vi "RT.vi"() -> ()   [LabVIEW 2020]
uses:
  <vilib>/FPGAPlugInAG/cRIO-9054/niLvFpga_Open_cRIO-9054.vi
  <vilib>/FPGAPlugInAG/cRIO-9054/niLvFpga_Reset_cRIO-9054.vi
  <vilib>/Utility/error.llb/Error Cluster From Error Code.vi
  <vilib>/rvi/errors/niLvFpgaAdjustHostInterfaceError.vi
  <vilib>/FPGAPlugInAG/cRIO-9054/niLvFpga_Run_cRIO-9054.vi
  <vilib>/FPGAPlugInAG/cRIO-9054/niLvFpga_Close_cRIO-9054.vi
  <vilib>/rvi/interface/nirviOpenFPGA/nirviOpenFPGA.xnode
  FPGA Bitfiles/fftwithlatch_FPGATarget_FPGA_RWnWaooWQ68.lvbitx
  FPGA.vi
  <vilib>/rvi/interface/nirviMethod/nirviMethod.xnode
  <vilib>/rvi/interface/nirviReadWriteControl/nirviReadWriteControl.xnode
  <vilib>/rvi/interface/nirviCloseFPGA/nirviCloseFPGA.xnode
  <vilib>/rvi/errors/niLvFpgaMergeErrorWithErrorCode.vi
  <vilib>/FPGAPlugInAG/cRIO-9054/niLvFpga_ReadFifo_cRIO-9054.vi
  NiFpgaLv.dll
  <vilib>/FPGAPlugInAG/cRIO-9054/niLvFpga_StartFifo_cRIO-9054.vi
panel:
  out "index":i32[](array[numeric])
  out "Index":i32[](graph)
  out "IMG":dbl[](graph)
  out "REAL":dbl[](graph)
  in  "FFT loop iterations":i32
  in  "auto stop":bool=TRUE
  out "FFT time (uSec)":u32
  out "data collection time (uSec)":u32
  in  "number of date points":i32=9000
  out "Timed Out?":bool
  in  "requested Loop rate (Hz)":u32=1000
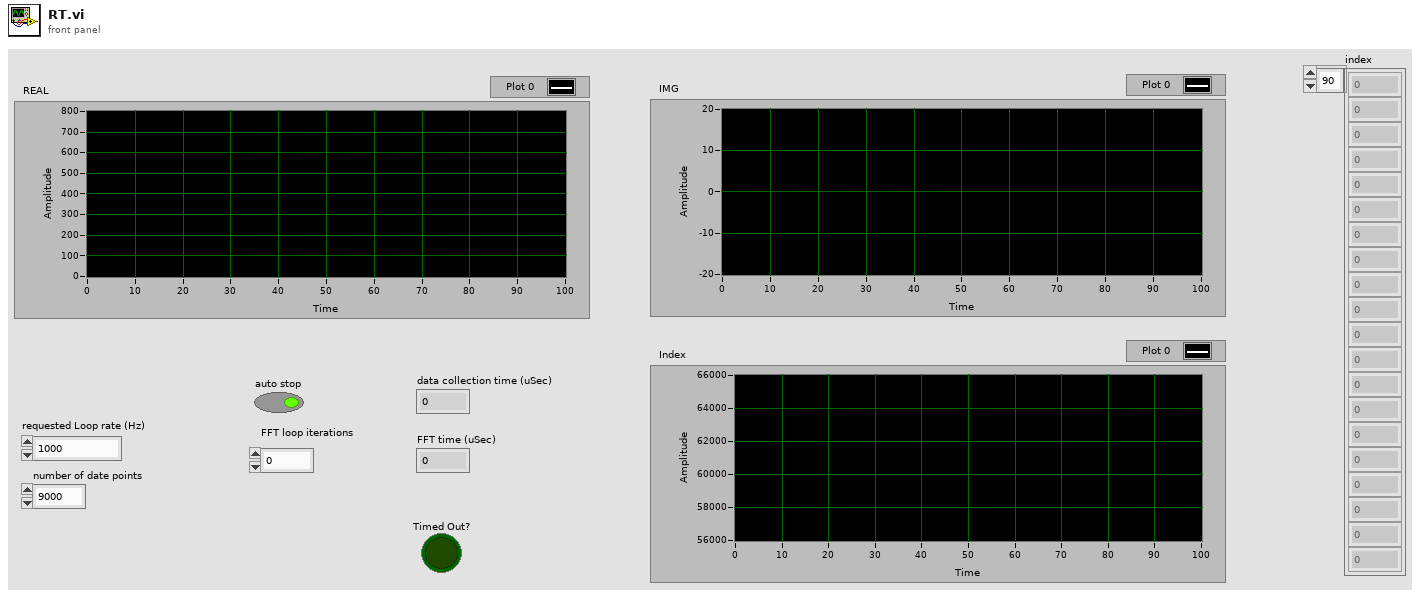
[diagram p1: front panel]
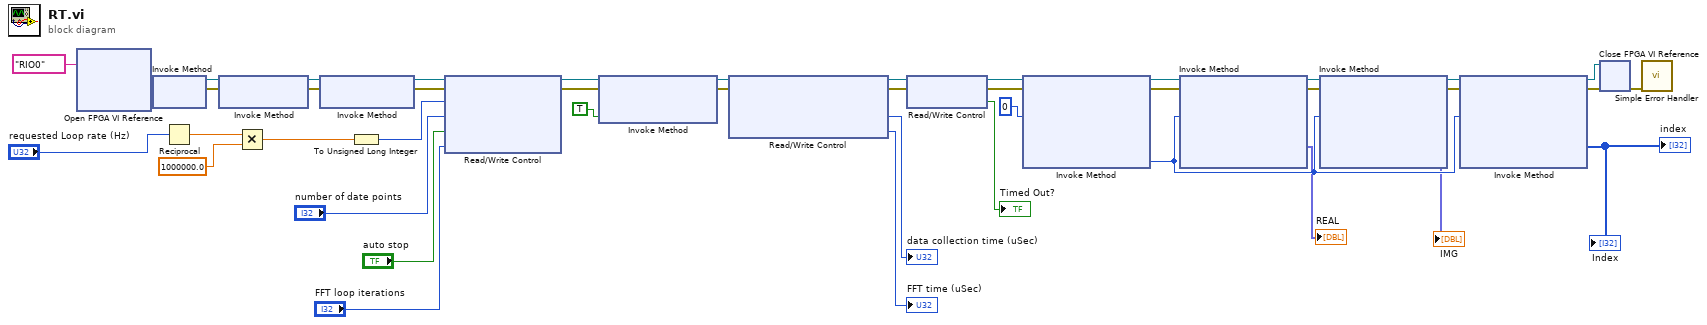
[diagram p0: block diagram]
diagram:
  n1 = xnode "Open FPGA VI Reference"("resource name"=tag "RIO0") -> ("FPGA VI Reference Out"=w23:refnum<k20>, "error out"=w22:errorcluster)  [unwired: 1 in]
  n2 = xnode "Invoke Method"("FPGA VI Reference In"=w23, "error in"=w22) -> ("FPGA VI Reference Out"=w16:refnum<k20>, "error out"=w15:errorcluster)
  n3 = Reciprocal(x="requested Loop rate (Hz)") -> (1/x=w37:dbl)
  n4 = xnode "Invoke Method"("FPGA VI Reference In"=w16, "error in"=w15) -> ("FPGA VI Reference Out"=w18:refnum<k20>, "error out"=w17:errorcluster)
  n5 = Multiply(x=w37, y=1000000.0) -> (x*y=w35:dbl)
  n6 = xnode "Invoke Method"("FPGA VI Reference In"=w18, "error in"=w17) -> ("FPGA VI Reference Out"=w10:refnum<k20>, "error out"=w9:errorcluster)
  n7 = To Unsigned Long Integer(number=w35) -> (unsigned 32bit integer=w34:u32)
  n8 = xnode "Read/Write Control"("FPGA VI Reference In"=w10, "error in"=w9, "Rate (uSec)"=w34, "Loop number"="number of date points", "auto stop"="auto stop", "FFT loop iterations"="FFT loop iterations") -> ("FPGA VI Reference Out"=w43:refnum<k20>, "error out"=w42:errorcluster)
  n9 = xnode "Invoke Method"("FPGA VI Reference In"=w43, "error in"=w42, "Wait Until Done (F)"=TRUE) -> ("FPGA VI Reference Out"=w39:refnum<k20>, "error out"=w38:errorcluster)
  n10 = xnode "Read/Write Control"("FPGA VI Reference In"=w39, "error in"=w38) -> ("FPGA VI Reference Out"=w14:refnum<k20>, "error out"=w13:errorcluster, "data collection time (uSec)"=→"data collection time (uSec)":u32, "FFT time (uSec)"=→"FFT time (uSec)":u32)  [unwired: 1 out]
  n11 = xnode "Read/Write Control"("FPGA VI Reference In"=w14, "error in"=w13) -> ("FPGA VI Reference Out"=w12:refnum<k20>, "error out"=w11:errorcluster, "Timed Out?"=→"Timed Out?":bool)
  n12 = xnode "Invoke Method"("FPGA VI Reference In"=w12, "error in"=w11, "Number of Elements"=u32 0) -> ("FPGA VI Reference Out"=w29:refnum<k20>, "error out"=w28:errorcluster, "Elements Remaining"=w4:u32)  [unwired: 1 in, 1 out]
  n13 = xnode "Invoke Method"("FPGA VI Reference In"=w29, "error in"=w28, "Number of Elements"=w4) -> ("FPGA VI Reference Out"=w32:refnum<k20>, "error out"=w31:errorcluster, "Data"=→"REAL":fxp<+/-,32,21>[])  [unwired: 1 in, 1 out]
  n14 = xnode "Invoke Method"("FPGA VI Reference In"=w32, "error in"=w31, "Number of Elements"=w4) -> ("FPGA VI Reference Out"=w8:refnum<k20>, "error out"=w7:errorcluster, "Data"=→"IMG":fxp<+/-,32,21>[])  [unwired: 1 in, 1 out]
  n15 = xnode "Invoke Method"("FPGA VI Reference In"=w8, "error in"=w7, "Number of Elements"=w4) -> ("FPGA VI Reference Out"=w6:refnum<k20>, "error out"=w5:errorcluster, "Data"=→"Index" →"index":i32[])  [unwired: 1 in, 1 out]
  n16 = xnode "Close FPGA VI Reference"("FPGA VI Reference In"=w6, "error in"=w5) -> ("error out"=w33:errorcluster)
  n17 = call <vilib>:"Simple Error Handler.vi"("error in (no error)"=w33) -> ()  [unwired: 4 in, 5 out]
